vi "Data Buffer.vi"(6 "Data in":u32[][](array[numeric]), 7 "Operation":T1(ring), 9 "Samples to read":u32, 10 "Samples per channel":u32, 11 "Channels":i32) -> (1 "Elements remaining":u32, 4 "Data out":u32[][](array[numeric]))   [LabVIEW 2021]
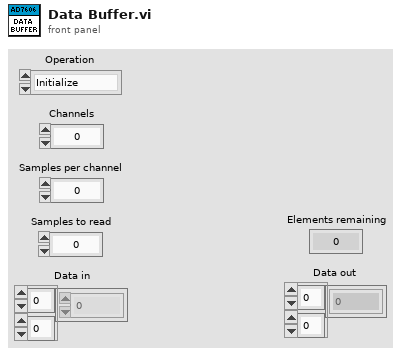
[diagram p1: front panel]
types:
  T1 = enum16{"Initialize", "Write", "Read", "GetBacklog", "Reset"}
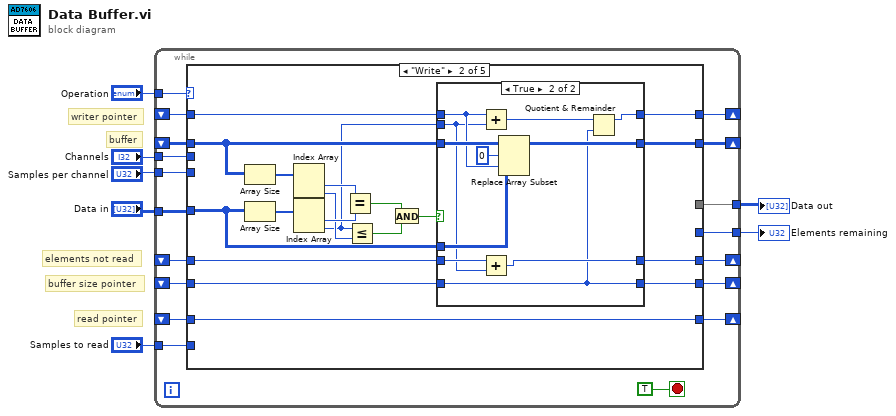
[diagram p0: block diagram]
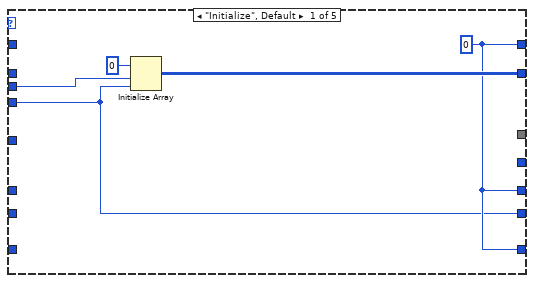
[diagram p2: hidden frame]
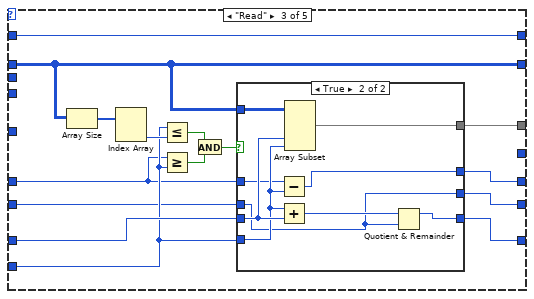
[diagram p4: hidden frame]
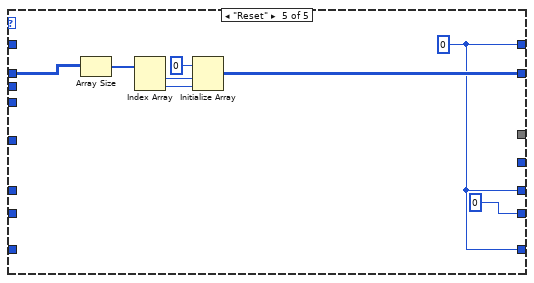
[diagram p7: hidden frame]
diagram:
  # "buffer size pointer"
  # "read pointer"
  # "elements not read"
  # "buffer"
  # "writer pointer"
  n1 = while {
    tunnel: "Operation" -> [w24]
    tunnel: "Channels" -> [w23]
    tunnel: "Samples per channel" -> [w22]
    shift-right: [w21] -> _
    shift-left: _ -> [w20]
    shift-right: [w10] -> _
    shift-left: _ -> [w9]
    tunnel: "Samples to read" -> [w19]
    shift-right: [w11] -> _
    shift-left: _ -> [w8]
    shift-right: [w18] -> _
    shift-left: _ -> [w17]
    tunnel: [w16] -> w2
    tunnel: [w15] -> w1
    tunnel: "Data in" -> [w14]
    shift-right: [w13] -> _
    shift-left: _ -> [w12]
    stop <- TRUE stop-if-true
    n2 = case shown="\"Write\"" w24 {
      tunnel: w23 -> [w29 _ _ _ _]
      tunnel: w22 -> [w26 _ _ _ _]
      tunnel: [w28 w39 w74 w95 w100] -> w21
      tunnel: w20 -> [_ w41 w74 w95 w99]
      tunnel: w14 -> [_ w40 _ _ _]
      tunnel: w9 -> [_ w38 w66 w96 _]
      tunnel: [w27 w36 w66 w96 w98] -> w10
      tunnel: w19 -> [_ _ w72 _ _]
      tunnel: [w27 w35 w70 w94 w98] -> w11
      tunnel: w8 -> [_ w35 w73 w94 _]
      tunnel: [w27 w33 w68 w93 w98] -> w18
      tunnel: w17 -> [_ w34 w69 w93 _]
      tunnel: [_ _ w71 _ _] -> w16
      tunnel: [_ _ _ w93 _] -> w15
      tunnel: [w26 w31 w67 w92 u32 0 ("Samples per channel")] -> w13
      tunnel: w12 -> [_ w32 w65 w92 _]
      frame "Initialize", Default {
        w27 = u32 0 ("disabled index (col)")
        n3 = Initialize Array(u32 0, w29, w26) -> (w28:u32[][])
      }
      frame "Write" {
        n4 = Array Size(array=w41) -> (size(s)=w48:i32[])
        n5 = Array Size(array=w40) -> (size(s)=w49:i32[])
        n6 = Index Array(array=w48) -> (element #1=w47:i32, element #2=w45:i32)  [unwired: 2 in]
        n7 = Index Array(array=w49) -> (element #1=w46:i32, element #2=w37:i32)  [unwired: 2 in]
        n8 = Equal?(x=w47, y=w46) -> (x = y?=w43:bool)
        n9 = Less Or Equal?(x=w37, y=w45) -> (x <= y?=w44:bool)
        n10 = And(x=w43, y=w44) -> (x .and. y?=w42:bool)
        n11 = case shown="True" w42 {
          tunnel: w41 -> [w53 w64]
          tunnel: w40 -> [_ w61]
          tunnel: [w53 w63] -> w39
          tunnel: w38 -> [w52 w60]
          tunnel: w37 -> [_ w58]
          tunnel: [w52 w54] -> w36
          tunnel: w34 -> [w51 w59]
          tunnel: [w51 w57] -> w33
          tunnel: w32 -> [w50 w55]
          tunnel: [w50 w55] -> w31
          frame False {
          }
          frame True {
            n12 = Add(x=w60, y=w58) -> (x+y=w56:u32)
            n13 = Add(x=w59, y=w58) -> (x+y=w57:u32)
            n14 = Replace Array Subset(array=w64, new element=w61, index (row)=0 ("disabled index (row)"), index (col)=w60) -> (w63:u32[][])
            n15 = Quotient & Remainder(x=w56, y=w55) -> (x-y*floor(x/y)=w54:u32)  [unwired: 1 out]
          }
        }
      }
      frame "Read" {
        n16 = Array Size(array=w74) -> (size(s)=w79:i32[])
        n17 = Index Array(array=w79) -> (element #2=w78:i32)  [unwired: 2 in, 1 out]
        n18 = Less Or Equal?(x=w72, y=w78) -> (x <= y?=w77:bool)
        n19 = Greater Or Equal?(x=w69, y=w72) -> (x >= y?=w76:bool)
        n20 = And(x=w77, y=w76) -> (x .and. y?=w75:bool)
        n21 = case shown="True" w75 {
          tunnel: w74 -> [_ w91]
          tunnel: w73 -> [w82 w89]
          tunnel: w72 -> [_ w88]
          tunnel: [_ w90] -> w71
          tunnel: [w82 w84] -> w70
          tunnel: w69 -> [w81 w87]
          tunnel: [w81 w86] -> w68
          tunnel: w65 -> [w80 w83]
          tunnel: [w80 w83] -> w67
          frame False {
          }
          frame True {
            n22 = Subtract(x=w87, y=w88) -> (x-y=w86:u32)
            n23 = Add(x=w88, y=w89) -> (x+y=w85:u32)
            n24 = Array Subset(array=w91, index (col)=w89, length (col)=w88) -> (w90:u32[][])  [unwired: 2 in]
            n25 = Quotient & Remainder(x=w85, y=w83) -> (x-y*floor(x/y)=w84:u32)  [unwired: 1 out]
          }
        }
      }
      frame "GetBacklog" {
      }
      frame "Reset" {
        w98 = u32 0 ("disabled index (col)")
        n26 = Array Size(array=w99) -> (size(s)=w104:i32[])
        n27 = Index Array(array=w104) -> (element #1=w102:i32, element #2=w103:i32)  [unwired: 2 in]
        n28 = Initialize Array(u32 0, w102, w103) -> (w100:u32[][])
      }
    }
  }
  "Elements remaining" <- w1
  "Data out" <- w2
